vi "S2DS_ConfigReadAdditionalInfo (SubVI).vi"(8 "error in (no error)":errorcluster, 10 "False channel (in) in":string[][](array[string]), 11 "file path (use dialog)":path) -> (0 "error out":errorcluster, 2 "False channel (in) out":string[][](array[string]))   [LabVIEW 2025]
uses:
  <vilib>/regexp/Match Regular Expression.xnode
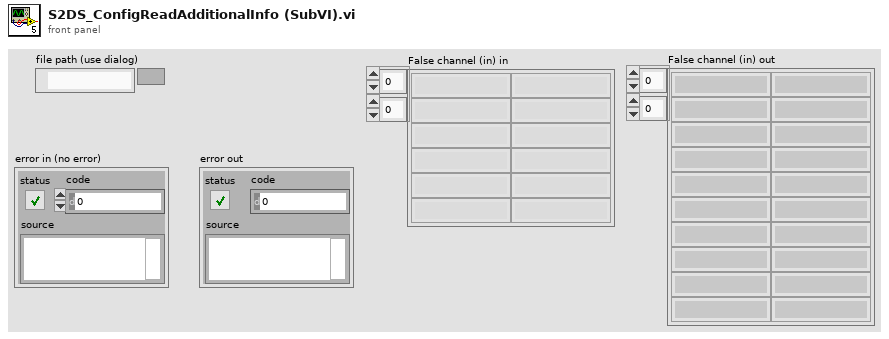
[diagram p1: front panel]
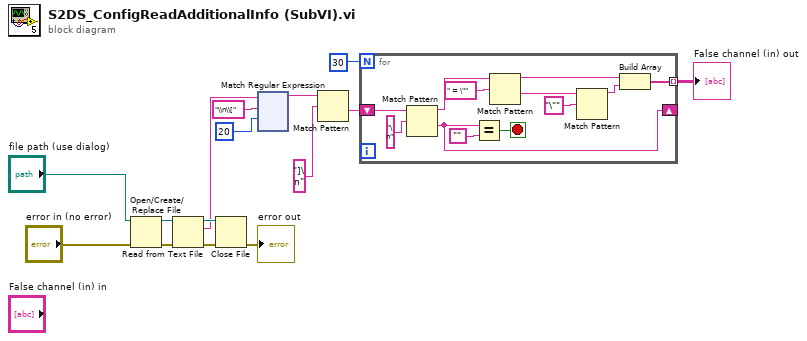
[diagram p0: block diagram]
diagram:
  n1 = Open/Create/Replace File(file path (use dialog)="file path (use dialog)", error in="error in (no error)") -> (refnum out=w13:refnum<file>, error out=w12:errorcluster)  [unwired: 4 in, 1 out]
  n2 = Read from Text File(file (use dialog)=w13, error in=w12) -> (refnum out=w10:refnum<file>, text=w2:string, error out=w11:errorcluster)  [unwired: 2 in, 1 out]
  n3 = Close File(refnum=w10, error in=w11) -> (error out=→"error out":errorcluster)  [unwired: 1 out]
  n4 = xnode "Match Regular Expression"("input string"=w2, "regular expression"="\\n\\[", "offset (0)"=20) -> ("before match"=w5:string)  [unwired: 3 in, 4 out]
  n5 = Match Pattern(string=w5, regular expression="]\n") -> (after substring=w3:string)  [unwired: 1 in, 3 out]
  n6 = for {
    N: 30 -> [_]
    shift-right: [w25] -> _
    shift-left: w3 -> [w27]
    tunnel: [w16] -> w1 mode=indexing
    stop <- w24 stop-if-true
    n7 = Match Pattern(string=w27, regular expression="\n") -> (before substring=w22:string, after substring=w25:string)  [unwired: 1 in, 2 out]
    n8 = Equal?(x=w25, y="") -> (x = y?=w24:bool)
    n9 = Match Pattern(string=w22, regular expression=" = \"") -> (before substring=w20:string, after substring=w19:string)  [unwired: 1 in, 2 out]
    n10 = Match Pattern(string=w19, regular expression="\"") -> (before substring=w17:string)  [unwired: 1 in, 3 out]
    n11 = Build Array(w20, w17) -> (w16:string[])
  }
  "False channel (in) out" <- w1
